vi "Cluster AutoSizing.vi"(6 "Variant in":variant, 7 "Shift Pressed?":bool, 8 "error in (no error)":errorcluster, 10 "QD Combo Box Ref":refnum<vi>, 11 "QD Launch VI Ref":refnum<vi>) -> (0 "error out":errorcluster, 4 "Variant out":variant)   [LabVIEW 2012, in "Cluster AutoSizing.lvlib"]
doc: "Using a float dialog to choose cluster auto-sizing type. Press `Shift` to set the contained cluster items recursively. \n\n- None\n- Size to Fit\n- Arrange Horizontally\n- Arrange Vertically\n\nDefault Shortcut - [U]"
uses:
  Cluster AutoSizing.lvlib
panel:
  in  "Undo Name":string="Cluster autosizing"
  # "Do not change the connector pane of this VI.\n\nSee the block diagram for directions on how to use this template."
  # "Specify the name of the Undo transaction"
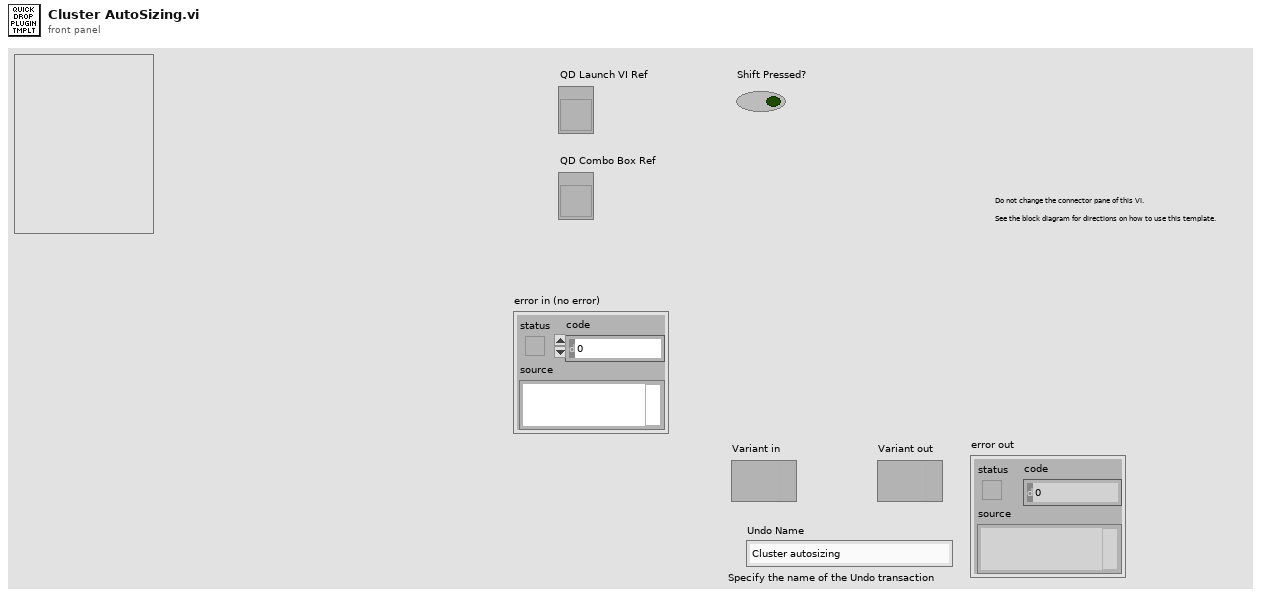
[diagram p1: front panel]
types:
  T1 = enum16{"None", "Size to Fit", "Arrange Horizontally", "Arrange Veritcally"}
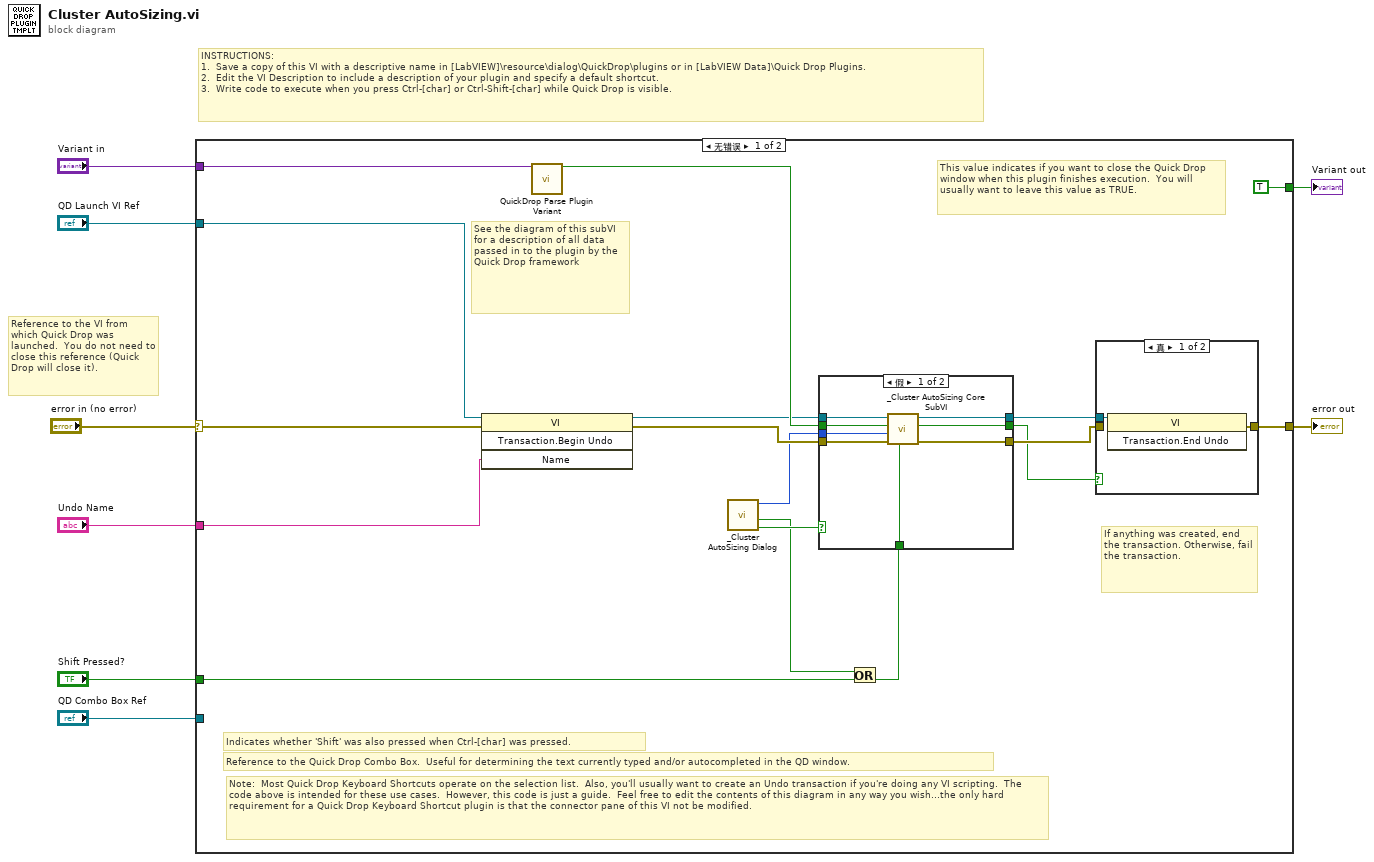
[diagram p0: block diagram]
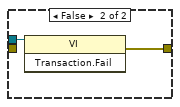
[diagram p3: hidden frame]
diagram:
  # "Reference to the VI from which Quick Drop was launched.  You do not need to close this reference (Quick Drop will close it)."
  # "INSTRUCTIONS:\n1.  Save a copy of this VI with a descriptive name in [LabVIEW]\\resource\\dialog\\QuickDrop\\plugins or in [LabVIEW Data]\\Quick Drop Plugins.\n2.  Edit the VI Description to include a description of your plugin and specify a default shortcut. \n3.  Write code to execute when you press Ctrl-[char] or Ctrl-Shift-[char] while Quick Drop is visible."
  n1 = case shown="无错误" "error in (no error)" {
    selector: "error in (no error)" -> [w24 w40]
    tunnel: [w18 w40] -> w8
    tunnel: "QD Launch VI Ref" -> [w23 _]
    tunnel: "Shift Pressed?" -> [w11 _]
    tunnel: "QD Combo Box Ref" -> [_ _]
    tunnel: "Variant in" -> [w25 _]
    tunnel: "Undo Name" -> [w22 _]
    tunnel: [TRUE _] -> w2
    frame No Error {
      # "Note:  Most Quick Drop Keyboard Shortcuts operate on the selection list.  Also, you'll usually want to create an Undo transaction if you're doing any VI scripting.  The code above is intended for these use cases.  However, this code is just a guide.  Feel free to edit the contents of this diagram in any way you wish...the only hard requirement for a Quick Drop Keyboard Shortcut plugin is that the connector pane of this VI not be modified."
      # "If anything was created, end the transaction. Otherwise, fail the transaction."
      # "This value indicates if you want to close the Quick Drop window when this plugin finishes execution.  You will usually want to leave this value as TRUE."
      # "See the diagram of this subVI for a description of all data passed in to the plugin by the Quick Drop framework"
      # "Reference to the Quick Drop Combo Box.  Useful for determining the text currently typed and/or autocompleted in the QD window."
      # "Indicates whether 'Shift' was also pressed when Ctrl-[char] was pressed."
      n2 = invoke class="VI" method="Transaction.Begin Undo"(reference=w23, error in=w24, "Name"=w22) -> (reference out=w14:refnum<vi>, error out=w19:errorcluster)  [unwired: 1 in, 2 out]
      n3 = call <vilib>:"QuickDrop Parse Plugin Variant.vi"("QDKS Variant in"=w25) -> ("QD Launch VI Panel?"=w20:bool)  [unwired: 12 in, 2 out]
      n4 = call "_Cluster AutoSizing Dialog.vi"() -> ("cancelled?"=w12:bool, "Recursively (dup)"=w9:bool, "type"=w16:T1)  [unwired: 9 in]
      n5 = Or(x=w9, y=w11) -> (x .or. y?=w10:bool)
      n6 = case shown="假" w12 {
        tunnel: w20 -> [w33 _]
        tunnel: w19 -> [w32 w34]
        tunnel: [w31 w34] -> w17
        tunnel: w16 -> [w30 _]
        tunnel: [w29 _] -> w15
        tunnel: w14 -> [w28 w35]
        tunnel: [w27 w35] -> w13
        tunnel: w10 -> [w26 _]
        frame False {
          n7 = call "_Cluster AutoSizing Core SubVI.vi"("recursive"=w26, "error in (no error)"=w32, "type"=w30, "QD Launch VI Panel?"=w33, "VI in"=w28) -> ("error out"=w31:errorcluster, "Changed?"=w29:bool, "VI out"=w27:refnum<vi>)  [unwired: 4 in]
        }
        frame True {
        }
      }
      n8 = case shown="真" w15 {
        tunnel: w13 -> [w36 w38]
        tunnel: [w37 w39] -> w18
        tunnel: w17 -> [_ _]
        frame True {
          n9 = invoke class="VI" method="Transaction.End Undo"(reference=w36) -> (error out=w37:errorcluster)  [unwired: 2 in, 2 out]
        }
        frame False {
          n10 = invoke class="VI" method="Transaction.Fail"(reference=w38) -> (error out=w39:errorcluster)  [unwired: 2 in, 2 out]
        }
      }
    }
    frame Error {
    }
  }
  "error out" <- w8
  "Variant out" <- w2
